vi "ComboBox.vi"() -> ()   [LabVIEW 2018]
panel:
  out "Selected Day":string
  in  "Combo Box":string(combo)="Sunday"
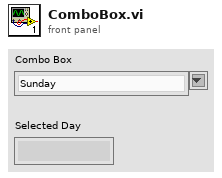
[diagram p1: front panel]
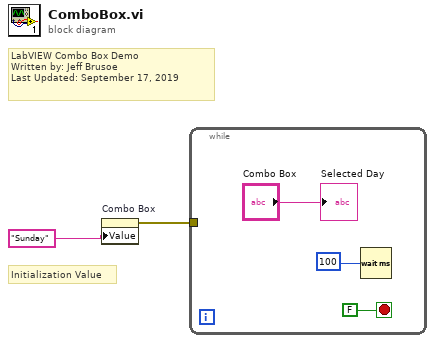
[diagram p0: block diagram]
diagram:
  # "Initialization Value"
  # "LabVIEW Combo Box Demo\nWritten by: Jeff Brusoe\nLast Updated: September 17, 2019"
  n1 = property on="Combo Box" class="CmbBox"("Value"="Sunday") -> (error out=w2:errorcluster)  [unwired: 2 in, 1 out]
  n2 = while {
    tunnel: w2 -> [_]
    stop <- FALSE stop-if-true
    n3 = Wait (ms)(milliseconds to wait=u32 100) -> ()  [unwired: 1 out]
    "Selected Day" <- "Combo Box"
  }
